vi "Main.vi"() -> ()   [LabVIEW 2016]
uses:
  <vilib>/Platform/TimedLoop/XDataNode/timing_clust.ctl
  <vilib>/Platform/TimedLoop/XDataNode/nitl_modes.ctl
  <vilib>/Platform/TimedLoop/XDataNode/wakeup.ctl
  Globale Variable/Globale Variable.vi
  <vilib>/Platform/TimedLoop/XDataNode/XDataNode.xnode
  <vilib>/Platform/TimedLoop/XDataNode/XDNodeRunTimeDep.lvlib
panel:
  in  "R":dbl
  in  "Q":dbl
  in  "LAUNCH":bool
  in  "Manual Gain":bool
  in  "voltage_start":dbl
  in  "starting threshold":dbl
  in  "v_max":dbl
  in  "k_lqr":dbl
  out "error out":errorcluster
  in  "lambda_target":dbl=0.1
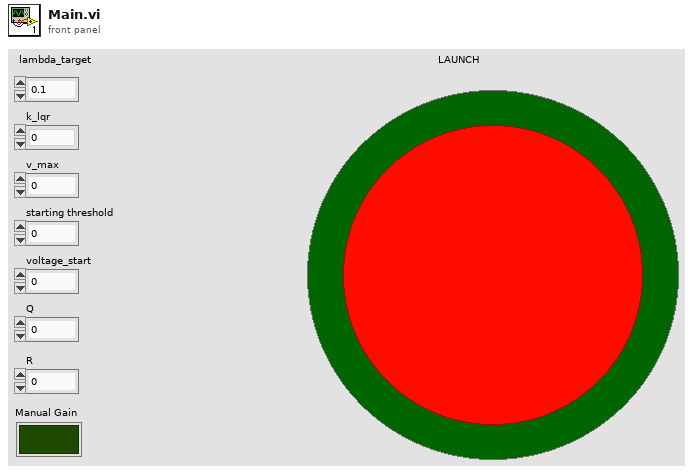
[diagram p1: front panel]
types:
  T1 = typedef "XDNodeRunTimeDep.lvlib/timing_clust.ctl" = cluster{"Expected End [f-1]":u64, "Actual End [f-1]":u64, "Finished Late? [f-1]":bool, "Expected End [i-1]":u64, "Actual End [i-1]":u64, "Finished Late? [i-1]":bool, "Expected Start [i]":u64, "Actual Start [i]":u64, "Expected Start [f]":u64, "Actual Start [f]":u64, "Source Name":string, "Structure Name":string, "Period":i64, "Deadline":i64, "Offset":i64, "Start":i64, "Priority":i32, "Timeout":i32, "Mode":T2, "Wakeup Reason":T3, "Error":errorcluster, "Source Type":string, "Secondary Source Type":string, "Global End Time":u64, "Global Start Time":u64, "Frame Duration":u64, "Iteration Duration":u64, "Assigned CPU":i32, "I/O Scan Engine Mode":u32}
  T2 = typedef "XDNodeRunTimeDep.lvlib/nitl_modes.ctl" = enum32{"No Change", "Process missed periods, maintain original phase", "Discard missed periods, maintain original phase", "Process missed periods, ignore original phase", "Discard missed periods, ignore original phase"}
  T3 = typedef "XDNodeRunTimeDep.lvlib/wakeup.ctl" = enum32{"Normal", "Aborted", "Asynchronous wakeup", "Timing source error", "Timed loop error", "Timeout"}
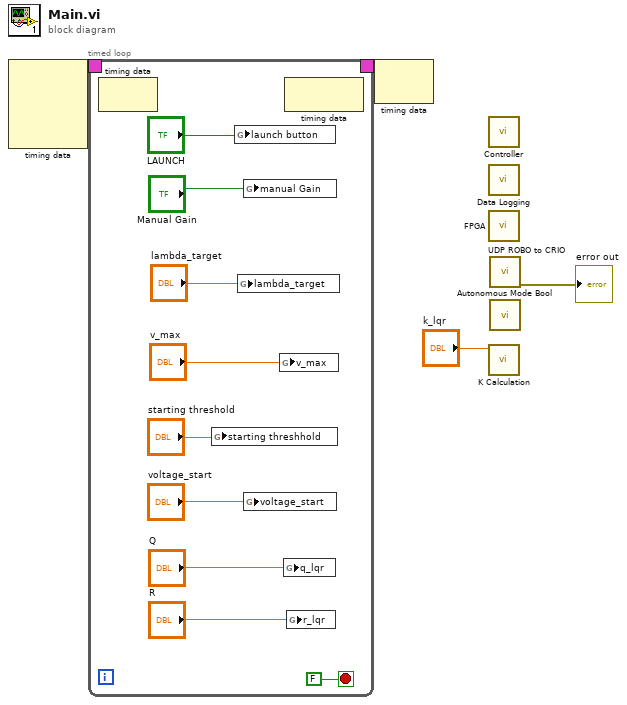
[diagram p0: block diagram]
diagram:
  n1 = node-c288() -> (w2:T1)  [unwired: 4 in]
  n2 = timed-loop {
    timing: w2 -> [_]
    timing-out: [_] -> w1
    stop <- FALSE stop-if-true
    n3 = node-c288() -> ()  [unwired: 1 in, 1 out]
    n4 = global write "Globale Variable.vi" "starting threshhold"("starting threshold") -> ()
    n5 = global write "Globale Variable.vi" "launch button"("LAUNCH") -> ()
    n6 = global write "Globale Variable.vi" "lambda_target"("lambda_target") -> ()
    n7 = global write "Globale Variable.vi" "manual Gain"("Manual Gain") -> ()
    n8 = global write "Globale Variable.vi" "voltage_start"("voltage_start") -> ()
    n9 = global write "Globale Variable.vi" "v_max"("v_max") -> ()
    n10 = global write "Globale Variable.vi" "q_lqr"("Q") -> ()
    n11 = node-c288() -> ()  [unwired: 1 in, 1 out]
    n12 = global write "Globale Variable.vi" "r_lqr"("R") -> ()
  }
  n13 = node-c288(w1) -> ()  [unwired: 1 out]
  n14 = call "Controller.vi"() -> ()  [unwired: 12 in]
  n15 = call "Data Logging.vi"() -> ()  [unwired: 2 in]
  n16 = call "FPGA.vi"() -> ()  [unwired: 12 in]
  n17 = call "K Calculation.vi"("k_lqr"="k_lqr") -> ()  [unwired: 11 in]
  n18 = call "UDP ROBO to CRIO.vi"() -> ("error out"=→"error out":errorcluster)  [unwired: 11 in]
  n19 = call "Autonomous Mode Bool.vi"() -> ()  [unwired: 12 in]
